vi "logic_mux.vi"(2 "Control":T4, 3 "Input_results":T5, 4 "Input_flags":T1) -> (0 "Flags":T2, 1 "Result":T3)   [LabVIEW 2013]
panel:
  # "R1"
  # "R1"
  # "R1"
  # "R1"
  # "R1"
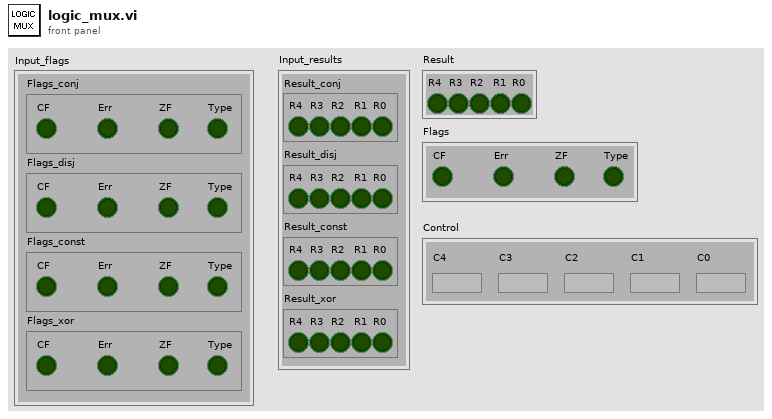
[diagram p1: front panel]
types:
  T1 = cluster{"Flags_conj":cluster{"CF":bool, "Err":bool, "ZF":bool, "Type":bool}, "Flags_disj":cluster{"CF":bool, "Err":bool, "ZF":bool, "Type":bool}, "Flags_const":cluster{"CF":bool, "Err":bool, "ZF":bool, "Type":bool}, "Flags_xor":cluster{"CF":bool, "Err":bool, "ZF":bool, "Type":bool}}
  T2 = cluster{"CF":bool, "Err":bool, "ZF":bool, "Type":bool}
  T3 = cluster{"R4":bool, "R3":bool, "R2":bool, bool, "R0":bool}
  T4 = cluster{"C4":bool, "C3":bool, "C2":bool, "C1":bool, "C0":bool}
  T5 = cluster{"Result_conj":cluster{"R4":bool, "R3":bool, "R2":bool, bool, "R0":bool}, "Result_disj":cluster{"R4":bool, "R3":bool, "R2":bool, bool, "R0":bool}, "Result_const":cluster{"R4":bool, "R3":bool, "R2":bool, bool, "R0":bool}, "Result_xor":cluster{"R4":bool, "R3":bool, "R2":bool, bool, "R0":bool}}
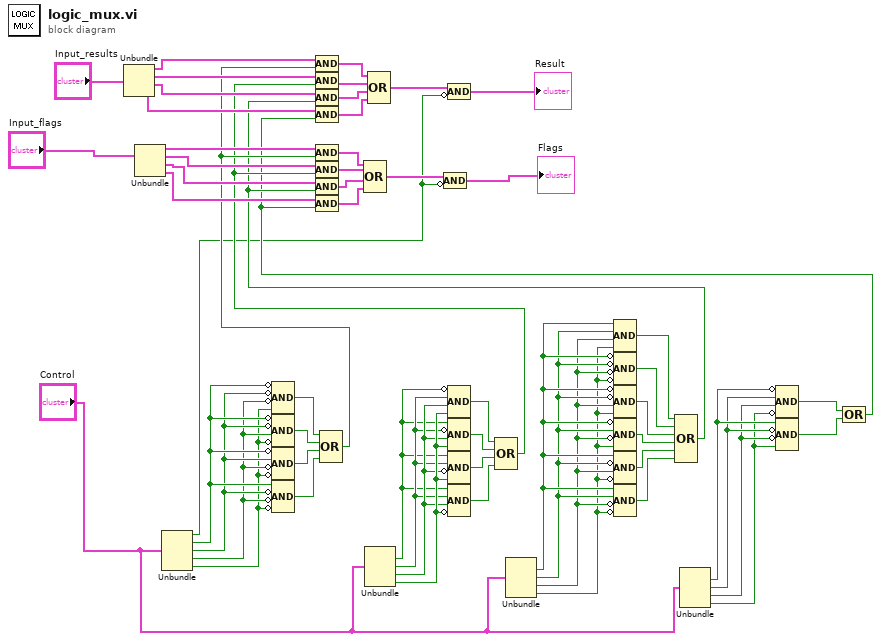
[diagram p0: block diagram]
diagram:
  n1 = Unbundle("Input_results") -> ("Result_conj"=w32:T3, "Result_disj"=w31:T3, "Result_const"=w30:T3, "Result_xor"=w29:T3)
  n2 = Unbundle("Input_flags") -> ("Flags_conj"=w28:T2, "Flags_disj"=w25:T2, "Flags_const"=w26:T2, "Flags_xor"=w27:T2)
  n3 = Unbundle("Control") -> ("C4"=w9:bool, "C3"=w58:bool, "C2"=w57:bool, "C1"=w56:bool, "C0"=w55:bool)
  n4 = Compound Arithmetic op=AND(invert w58, invert w57, invert w56, w55) -> (w46:bool)
  n5 = Compound Arithmetic op=AND(invert w58, invert w57, w56, invert w55) -> (w45:bool)
  n6 = Compound Arithmetic op=AND(invert w58, w57, invert w56, invert w55) -> (w43:bool)
  n7 = Compound Arithmetic op=AND(w58, invert w57, invert w56, invert w55) -> (w44:bool)
  n8 = Compound Arithmetic op=OR(w46, w45, w43, w44) -> (w24:bool)
  n9 = Compound Arithmetic op=AND(w32, w24) -> (w20:T3)
  n10 = Compound Arithmetic op=AND(w28, w24) -> (w16:T2)
  n11 = Unbundle("Control") -> ("C3"=w51:bool, "C2"=w52:bool, "C1"=w53:bool, "C0"=w54:bool)  [unwired: 1 out]
  n12 = Compound Arithmetic op=AND(invert w51, w52, w53, w54) -> (w42:bool)
  n13 = Compound Arithmetic op=AND(w51, invert w52, w53, w54) -> (w39:bool)
  n14 = Compound Arithmetic op=AND(w51, w52, invert w53, w54) -> (w40:bool)
  n15 = Compound Arithmetic op=AND(w51, w52, w53, invert w54) -> (w41:bool)
  n16 = Compound Arithmetic op=OR(w42, w39, w40, w41) -> (w23:bool)
  n17 = Compound Arithmetic op=AND(w31, w23) -> (w17:T3)
  n18 = Compound Arithmetic op=AND(w25, w23) -> (w13:T2)
  n19 = Unbundle("Control") -> ("C3"=w8:bool, "C2"=w7:bool, "C1"=w6:bool, "C0"=w5:bool)  [unwired: 1 out]
  n20 = Compound Arithmetic op=AND(w8, w7, w6, w5) -> (w3:bool)
  n21 = Compound Arithmetic op=AND(invert w8, invert w7, invert w6, invert w5) -> (w4:bool)
  n22 = Compound Arithmetic op=AND(invert w8, invert w7, w6, w5) -> (w38:bool)
  n23 = Compound Arithmetic op=AND(invert w8, w7, invert w6, w5) -> (w35:bool)
  n24 = Compound Arithmetic op=AND(w8, invert w7, w6, invert w5) -> (w36:bool)
  n25 = Compound Arithmetic op=AND(w8, w7, invert w6, invert w5) -> (w37:bool)
  n26 = Compound Arithmetic op=OR(w3, w4, w38, w35, w36, w37) -> (w22:bool)
  n27 = Compound Arithmetic op=AND(w30, w22) -> (w18:T3)
  n28 = Compound Arithmetic op=AND(w26, w22) -> (w14:T2)
  n29 = Unbundle("Control") -> ("C3"=w50:bool, "C2"=w49:bool, "C1"=w48:bool, "C0"=w47:bool)  [unwired: 1 out]
  n30 = Compound Arithmetic op=AND(invert w50, w49, w48, invert w47) -> (w34:bool)
  n31 = Compound Arithmetic op=AND(w50, invert w49, invert w48, w47) -> (w33:bool)
  n32 = Compound Arithmetic op=OR(w34, w33) -> (w21:bool)
  n33 = Compound Arithmetic op=AND(w29, w21) -> (w19:T3)
  n34 = Compound Arithmetic op=AND(w27, w21) -> (w15:T2)
  n35 = Compound Arithmetic op=OR(w16, w13, w14, w15) -> (w11:T2)
  n36 = Compound Arithmetic op=OR(w20, w17, w18, w19) -> (w12:T3)
  n37 = Compound Arithmetic op=AND(w11, invert w9) -> (→"Flags":T2)
  n38 = Compound Arithmetic op=AND(w12, invert w9) -> (→"Result":T3)
